vi "Transfer.vi"(5 "To Binding":refnum<class "Binding.lvclass">, 7 "From Binding":refnum<class "Binding.lvclass">, 8 "error in (no error)":errorcluster, 9 "To Class in":refnum<class>, 10 "From Class in":refnum<class>) -> (0 "error out":errorcluster, 1 "To Class out":refnum<class>, 2 "From Class out":refnum<class>)   [LabVIEW 2020, in "PropertyBinder.lvlib" / "Binding.lvclass"]
uses:
  Binding.lvclass
  Binding.lvclass/Binding.ctl
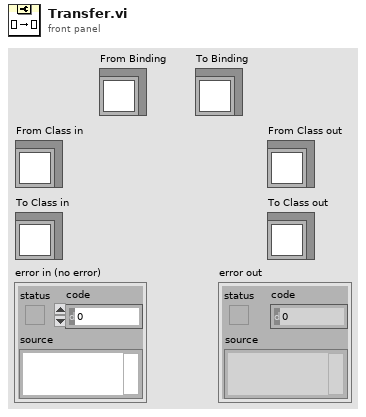
[diagram p1: front panel]
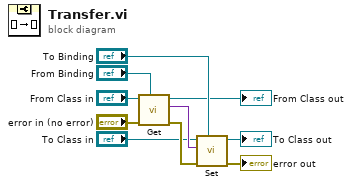
[diagram p0: block diagram]
diagram:
  n1 = call "Get.vi"("Binding"="From Binding", "error in (no error)"="error in (no error)", "Class in"="From Class in") -> ("error out"=w10:errorcluster, "Value"=w9:variant, "Class out"=→"From Class out":refnum<class>)  [unwired: 6 in]
  n2 = call "Set.vi"("Binding"="To Binding", "error in (no error)"=w10, "Value"=w9, "Class in"="To Class in") -> ("error out"=→"error out":errorcluster, "Class out"=→"To Class out":refnum<class>)  [unwired: 6 in]
